vi "DefaultPersonality_5785_FPGA.vi"() -> ()   [LabVIEW 2018, in "GettingStarted_5785_FPGA.lvlib"]
uses:
  GettingStarted_5785_FPGA.lvlib
  <instrlib>/_niInstr/Streaming/v1/Common/Stream State.ctl
  <vilib>/Platform/TimedLoop/XDataNode/timing_clust.ctl
  <vilib>/Platform/TimedLoop/XDataNode/nitl_modes.ctl
  <vilib>/Platform/TimedLoop/XDataNode/wakeup.ctl
  <instrlib>/FlexRIO/DRAM FIFO/v2/FPGA/DRAM FIFO/FIFO Depth.ctl
  <instrlib>/FlexRIO/API/FPGA/v1/IO/NI5785/AO DSP Cfg.ctl
  Generation Engine Cfg.ctl
  DDC Cfg.ctl
  <vilib>/rvi/Emulation/niFpgaSctlEmulationGetInTimedLoop.vi
  <vilib>/rvi/Emulation/niFpgaEmulationReportErrorSimple.vi
  <vilib>/rvi/Emulation/niFpgaGetClockAttributes.vi
  <vilib>/rvi/Emulation/niFpgaCriticalErrorInLSC.vi
  <vilib>/rvi/eio/common/nirviEmuTemplateMethod_errors.vi
  <vilib>/rvi/DataTransferAndStorage/Container/Common/niFpgaContainerGetUniqueNameForEmu.vi
  <vilib>/rvi/DataTransferAndStorage/Container/Common/niFpgaContainerSetEmuInfo.vi
  <vilib>/rvi/eio/common/nirviEmuReportErrorAndStop.vi
  <vilib>/rvi/interface/RandomDataEmulation/nirviRandomDataMultiElementFPGAFIFO.vi
  <instcachedir>/0/nirviRandomDataMultiElementFPGAFIFO_6740B454F3C245F78F76ED91F73FD8DB.lvgen/nirviRandomDataMultiElementFPGAFIFO_6740B454F3C245F78F76ED91F73FD8DB_002.vi
  <vilib>/rvi/interface/RandomDataEmulation/niFpgaRandomDataHandleErrors.vi
  <vilib>/rvi/DataTransferAndStorage/Container/Common/niFpgaContainerExecOnDevCompGetState.vi
  <vilib>/rvi/Emulation/niFpgaEmulationIsFPGAContextNoSignature.vi
  <vilib>/rvi/errors/niFpgaSetErrorForExecOnDevCompSimple.vi
  <vilib>/rvi/FIFO/Fifo_Resource/nirvififoEmulationSetSize.vi
  <vilib>/rvi/FIFO/Fifo_Resource/nirviFifoEmulationQueueMgr.vi
  <instcachedir>/0/nirviFifoEmulationQueueMgr_E5CAEC123FF24DC58D834DCA3CDAA9B5.lvgen/nirviFifoEmulationQueueMgr_E5CAEC123FF24DC58D834DCA3CDAA9B5_015.vi
  <vilib>/rvi/FIFO/Fifo_Resource/nirvififoEmulationDetermineInputValidOut.vi
  <vilib>/rvi/FIFO/Fifo_Resource/nirvififoEmulationCreateLock.vi
  <vilib>/rvi/Emulation/niFpgaProcessEmulError.vi
  <vilib>/rvi/FIFO/Fifo_Resource/nirvififoEmulationObtainLock.vi
  <vilib>/rvi/FIFO/Fifo_Resource/nirvififoEmulationReleaseLock.vi
  <vilib>/rvi/occurrence/nirviWaitOnOccurrenceBase.vi
  <vilib>/rvi/errors/nirviReportUnexpectedCaseInternalError.vi
  <vilib>/rvi/errors/nirviReportUnexpectedCaseInternalError (U32).vi
  <vilib>/Utility/error.llb/Clear Errors.vi
  <instrlib>/FlexRIO/DRAM FIFO/v2/FPGA/DRAM FIFO/Private/DRAM FIFO U256x2/Create 256x2 DRAM FIFO.vi
  <instrlib>/_niInstr/Data Formatting/v1/FPGA/Private/Convert/Boolean Array to U16 Array.vi
  <vilib>/Platform/TimedLoop/XDataNode/XDataNode.xnode
  <vilib>/eio/EIONode/EIONode.xnode
  <vilib>/rvi/LocalResourceManager/LocalResourceManager.xnode
  <vilib>/rvi/DataTransferAndStorage/Container/XNode/niFpgaContainer.xnode
  <vilib>/rvi/interface/RandomDataEmulation/nirviRandomDataFpgaMultiElementTemplate.vi
  <vilib>/rvi/FIFO/Fifo_Resource/niFpgaFifoEmulationRefIn.vi
  <vilib>/rvi/DataTransferAndStorage/Handshake/Emulation/niFpgaHandshakeEmulationRefIn.vi
  <vilib>/Platform/TimedLoop/XDataNode/XDNodeRunTimeDep.lvlib
  <instrlib>/FlexRIO/API/FPGA/v1/FlexRIO API FPGA v1.lvlib
  <instrlib>/FlexRIO/DRAM FIFO/v2/FPGA/DRAM FIFO/DRAM FIFO v2 FPGA.lvclass
  <instrlib>/_niInstr/Data Formatting/v1/FPGA/niInstr Data Formatting v1 FPGA.lvlib
  <instrlib>/FlexRIO/API/FPGA/v1/IO/NI5785/FlexRIO 5785 FPGA v1.lvlib
  <instrlib>/_niInstr/Streaming/v1/Common/niInstr Streaming v1 Common.lvlib
  <instrlib>/FlexRIO/DRAM FIFO/v2/FPGA/DRAM FIFO/Private/DRAM FIFO U256x2/DRAM FIFO U256x2 v2 FPGA.lvclass
panel:
  in  "flexrio.dsp.reset 1":bool
  in  "flexrio.stream.channels enabled 1":u64
  out "flexrio.dsp.ready 1":bool
  in  "flexrio.stream.data.complex 1":bool
  in  "flexrio.dsp.duc.enable 1":bool
  in  "flexrio.dsp.duc.freq shift.mag 1.1":fxp<+/-,48,0>
  in  "flexrio.dsp.duc.freq shift.mag 1.0":fxp<+/-,48,0>
  in  "flexrio.dsp.ddc.enable 0":bool
  in  "flexrio.dsp.ddc.freq shift.mag 0.1":fxp<+/-,48,0>
  in  "flexrio.dsp.ddc.freq shift.mag 0.0":fxp<+/-,48,0>
  out "flexrio.dsp.ready 0":bool
  in  "flexrio.dsp.reset 0":bool
  in  "User-defined Start Trigger - AO":bool
  in  "flexrio.trigger.start.cfg 1":u16
  in  "flexrio.trigger.start.linked 1":bool
  out "flexrio.buffer.circular.written 1":u64
  out "flexrio.buffer.circular.size 1":u64
  in  "flexrio.io.interleaving factor 0":u16=1
  out "IO Socket\\AO Ready For Input":bool
  in  "stream.request state 1":T1
  in  "stream.num samples 1":u64
  out "stream.metadata 1":u64
  out "stream.samples transferred 1":u64
  out "stream.state 1":T1
  in  "flexrio.buffer.circular.reset 1":bool
  out "flexrio.module.dram ready 0":bool
  in  "flexrio.buffer.fifo.reset 0":bool
  out "flexrio.module.io ready 0":bool
  out "flexrio.module.io error 0":i32
  out "flexrio.module.data valid 0":bool
  in  "flexrio.stream.channels enabled 0":u64 caption="stream.num samples 0"
  in  "flexrio.buffer.delay.clocks 0":u16=1
  in  "flexrio.buffer.delay.reset 0":bool
  in  "flexrio.trigger.analog.edge.rising 0":bool=TRUE
  in  "flexrio.trigger.analog.edge.hysteresis 0":fxp<+/-,32,1>
  in  "flexrio.trigger.analog.edge.threshold 0":fxp<+/-,32,1>
  in  "User-defined Start Trigger - AI":bool
  in  "flexrio.trigger.start.cfg 0":u16
  in  "flexrio.trigger.analog.edge.channel 0":fxp<+,2,2> format="%#_4g"
  in  "stream.num samples 0":u64
  in  "stream.request state 0":T1
  out "stream.state 0":T1
  out "stream.samples transferred 0":u64
  out "stream.metadata 0":u64
  # "Data Path Configuration"
  # "AI Trigger Configuration"
  # "AI Stream Configuration"
  # "AO Stream Configuration"
  # "AI DSP Configuration"
  # "AO DSP Configuration"
  # "User-defined Controls"
  # "Module Status"
  # "AO Buffer Configuration"
  # "Device Utilization\n---------------------------\nTotal Slices: 86.1% (35694 out of 41460)\nSlice Registers: 31.8% (211112 out of 663360)\nSlice LUTs: 48.0% (159148 out of 331680)\nBlock RAMs: 40.5% (437 out of 1080)\nDSP48s: 32.1% (886 out of 2760)\n\nNote: Utilization numbers are for the KU060. Exact values will vary for other variants"
  # "AO Trigger Configuration"
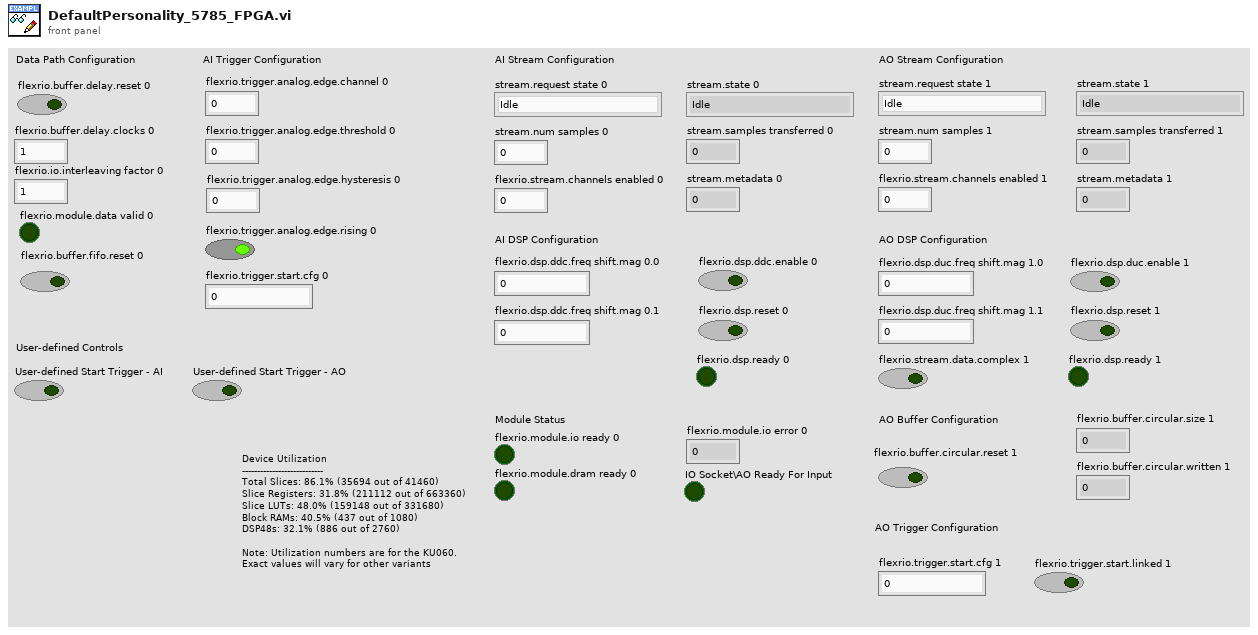
[diagram p1: front panel]
types:
  T1 = typedef "niInstr Streaming v1 Common.lvlib/Stream State.ctl" = enum8{"Idle", "Finite Transfer", "Continuous", "Done", "Error", "Not Ready", "Cancel"}
  T2 = typedef "XDNodeRunTimeDep.lvlib/timing_clust.ctl" = cluster{"Expected End [f-1]":u64, "Actual End [f-1]":u64, "Finished Late? [f-1]":bool, "Expected End [i-1]":u64, "Actual End [i-1]":u64, "Finished Late? [i-1]":bool, "Expected Start [i]":u64, "Actual Start [i]":u64, "Expected Start [f]":u64, "Actual Start [f]":u64, "Source Name":string, "Structure Name":string, "Period":i64, "Deadline":i64, "Offset":i64, "Start":i64, "Priority":i32, "Timeout":i32, "Mode":T3, "Wakeup Reason":T4, "Error":errorcluster, "Source Type":string, "Secondary Source Type":string, "Global End Time":u64, "Global Start Time":u64, "Frame Duration":u64, "Iteration Duration":u64, "Assigned CPU":i32, "I/O Scan Engine Mode":u32}
  T3 = typedef "XDNodeRunTimeDep.lvlib/nitl_modes.ctl" = enum32{"No Change", "Process missed periods, maintain original phase", "Discard missed periods, maintain original phase", "Process missed periods, ignore original phase", "Discard missed periods, ignore original phase"}
  T4 = typedef "XDNodeRunTimeDep.lvlib/wakeup.ctl" = enum32{"Normal", "Aborted", "Asynchronous wakeup", "Timing source error", "Timed loop error", "Timeout"}
  T5 = typedef "DRAM FIFO v2 FPGA.lvclass/FIFO Depth.ctl" = u8
  T6 = cluster{"flexrio.io.interleaving factor 0":u16, "flexrio.trigger.start.cfg 0":u16, "stream.num samples 0":u64, "stream.request state 0":T1, "flexrio.stream.channels enabled 0":u64, "flexrio.buffer.delay.clocks 0":u16, "flexrio.buffer.delay.reset 0":bool}
  T7 = typedef "GettingStarted_5785_FPGA.lvlib/DDC Cfg.ctl" = cluster{"flexrio.dsp.ddc.freq shift.mag 0.0":fxp<+/-,48,0>, "flexrio.dsp.ddc.freq shift.mag 0.1":fxp<+/-,48,0>, "flexrio.dsp.ddc.enable 0":bool, "flexrio.dsp.reset 0":bool}
  T8 = typedef "GettingStarted_5785_FPGA.lvlib/Generation Engine Cfg.ctl" = cluster{"flexrio.dsp.reset 1":bool, "flexrio.buffer.circular.reset 1":bool, "flexrio.stream.channels enabled 1":u64, "flexrio.trigger.start.linked 1":bool, "flexrio.trigger.start.cfg 1":u16, "stream.num samples 1":u64, "stream.request state 1":T1}
  T9 = cluster{"flexrio.trigger.analog.edge.channel 0":fxp<+,2,2>, "flexrio.trigger.analog.edge.threshold 0":fxp<+/-,32,1>, "flexrio.trigger.analog.edge.hysteresis 0":fxp<+/-,32,1>, "flexrio.trigger.analog.edge.rising 0":bool}
  T10 = typedef "FlexRIO 5785 FPGA v1.lvlib/AO DSP Cfg.ctl" = cluster{"flexrio.stream.data.complex 1":bool, "flexrio.dsp.duc.enable 1":bool, "flexrio.dsp.duc.freq shift.mag 1.0":fxp<+/-,48,0>, "flexrio.dsp.duc.freq shift.mag 1.1":fxp<+/-,48,0>}
  T11 = cluster{"stream.metadata 0":u64, "stream.samples transferred 0":u64, "stream.state 0":T1}
  T12 = cluster{"buffer size in elements":u64, "written elements":u64, "flexrio.dsp.ready 1":bool, "stream.metadata 1":u64, "stream.samples transferred 1":u64, "stream.state 1":T1}
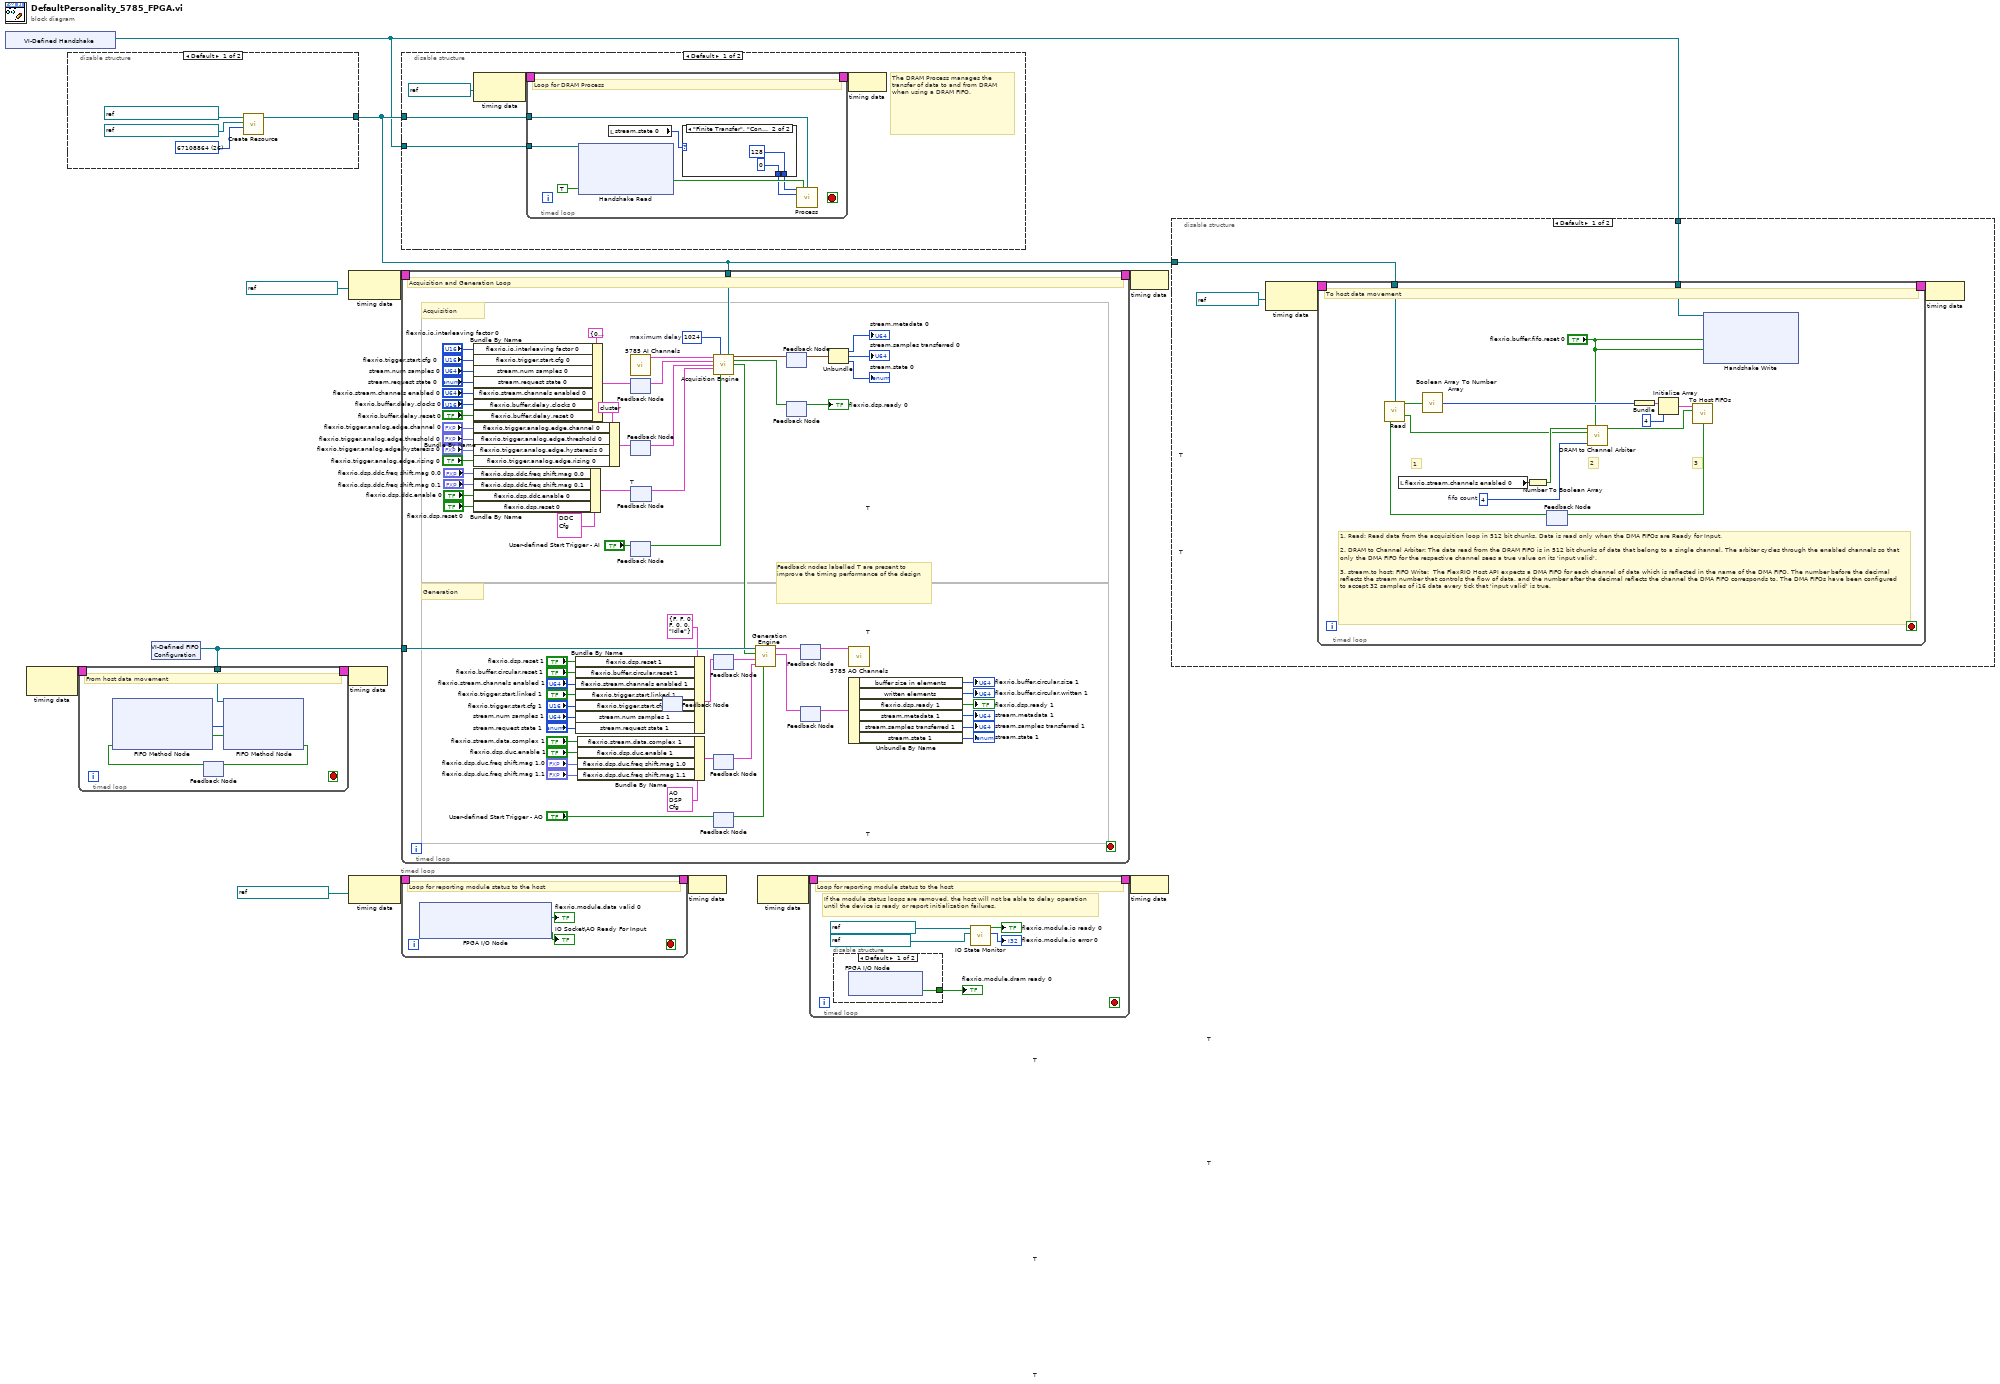
[diagram p0: block diagram]
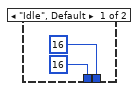
[diagram p3: hidden frame]
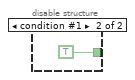
[diagram p6: hidden frame]
diagram:
  n1 = xnode "VI-Defined Handshake"() -> ("Handshake Out"=w7:refnum<k21>)
  n2 = node-c288() -> (w3:T2)  [unwired: 1 in]
  n3 = disable-structure shown="Default" {
    disable-tunnel: [w17 _] -> w8
    frame condition #0 (active) {
      w14 = T5 26 items=["4"=2, "8"=3, "16"=4, "32"=5, "64"=6, "128"=7, "256"=8, "512"=9, "1024"=10, "2048"=11, "4096"=12, "8192"=13, "16384"=14, "32768"=15, "65536"=16, "131072"=17, "262144"=18, "524288"=19, "1048576"=20, "2097152"=21, "4194304"=22, "8388608"=23, "16777216"=24, "33554432"=25, "67108864"=26, "134217728"=27, "268435456"=28, "536870912"=29, "1073741824"=30, "2147483648"=31, "4294967296"=32] ("actual # of DRAM elements")
      n4 = call-poly <instrlib>:"Create Resource.vi"("actual # of DRAM elements"=w14, "memory refnum 2"=refnum<k21> "DRAM FIFO Bank1 67108864" ("memory refnum"), "memory refnum"=refnum<k21> "DRAM FIFO Bank0 67108864") -> ("DRAM FIFO ref out"=w17:refnum<class "DRAM FIFO v2 FPGA.lvclass">)  [unwired: 8 in]
    }
    frame condition #1 {
    }
  }
  n5 = xnode "VI-Defined FIFO Configuration"() -> ("FIFO Out"=w1:refnum<k21>)
  n6 = timed-loop {
    timing: w3 -> [_]
    timing-out: [_] -> w2
    tunnel: w1 -> [w18]
    stop <- _ stop-if-true
    # "From host data movement"
    n7 = feedback #1() -> (w22:bool)  [unwired: 1 in]
    n8 = xnode ("FIFO Method Node")("Ready for Output"=w22) -> ("Element"=w19:i16[], "Output Valid"=w20:bool)  [unwired: 1 in, 1 out]
    n9 = xnode ("FIFO Method Node")("Element"=w19, "Input Valid"=w20, "FIFO In"=w18) -> ("Ready for Input"=w21:bool)  [unwired: 1 out]
    n10 = feedback-in #1(w21) -> ()
  }
  n11 = node-c288(refnum<k21> "IO Socket\\Data Clock" ("Source Name")) -> (w13:T2)
  n12 = node-c288(w2) -> ()
  n13 = node-c288(refnum<k21> "IO Socket\\Data Clock" ("Source Name")) -> (w6:T2)
  n14 = disable-structure shown="Default" {
    disable-tunnel: w8 -> [w26 _]
    disable-tunnel: w7 -> [w25 _]
    frame condition #0 (active) {
      # "The DRAM Process manages the transfer of data to and from DRAM when using a DRAM FIFO."
      n15 = node-c288(refnum<k21> "DRAM Clock" ("Source Name")) -> (w29:T2)
      n16 = timed-loop {
        timing: w29 -> [_]
        timing-out: [_] -> w28
        tunnel: w26 -> [w36]
        tunnel: w25 -> [w35]
        stop <- _ stop-if-true
        # "Loop for DRAM Process"
        n17 = xnode ("Handshake Read")("Ready for Output"=TRUE, "Handshake In"=w35) -> ("Output Valid"=w33:bool)  [unwired: 2 out]
        n18 = local read "stream.state 0"() -> (w32:T1)
        n19 = case shown="\"Finite Transfer\", \"Continuous\"" w32 {
          tunnel: [u16 16 ("write grant time (clock ticks)") u16 128 ("write grant time (clock ticks)")] -> w31
          tunnel: [u16 16 ("read grant time (clock ticks)") u16 0 ("read grant time (clock ticks)")] -> w30
          frame "Idle", Default {
          }
          frame "Finite Transfer", "Continuous" {
          }
        }
        n20 = call <instrlib>:"Process.vi"("write grant time (clock ticks)"=w31, "reset DRAM"=w33, "DRAM FIFO ref in"=w36, "read grant time (clock ticks)"=w30) -> ()  [unwired: 10 in, 2 out]
      }
      n21 = node-c288(w28) -> ()
    }
    frame condition #1 {
      # "The host can instruct the buffer to reset itself. To clear our all the data inside the FIFO the clear method is called. The clear method can only be accessed inside a while loop."
    }
  }
  n22 = timed-loop {
    timing: w13 -> [_]
    timing-out: [_] -> w12
    tunnel: w8 -> [w48]
    tunnel: w1 -> [w113]
    stop <- _ stop-if-true
    w47 = u16 1024  # maximum delay
    # "Feedback nodes labelled T are present to improve the timing performance of the design"
    # "Acquisition"
    # "Generation"
    # "Acquisition and Generation Loop"
    n23 = Bundle By Name(cluster=T6 {"flexrio.io.interleaving factor 0"=0, "flexrio.trigger.start.cfg 0"=0, "stream.num samples 0"=0, "stream.request state 0"=enum."Idle", "flexrio.stream.channels enabled 0"=0, "flexrio.buffer.delay.clocks 0"=0, "flexrio.buffer.delay.reset 0"=FALSE}, "flexrio.io.interleaving factor 0"="flexrio.io.interleaving factor 0", "flexrio.trigger.start.cfg 0"="flexrio.trigger.start.cfg 0", "stream.num samples 0"="stream.num samples 0", "stream.request state 0"="stream.request state 0", "flexrio.stream.channels enabled 0"="flexrio.stream.channels enabled 0", "flexrio.buffer.delay.clocks 0"="flexrio.buffer.delay.clocks 0", "flexrio.buffer.delay.reset 0"="flexrio.buffer.delay.reset 0") -> (w62:T6)
    n24 = Bundle By Name(cluster=T9 {"flexrio.trigger.analog.edge.channel 0"=0.0, "flexrio.trigger.analog.edge.threshold 0"=0.0, "flexrio.trigger.analog.edge.hysteresis 0"=0.0, "flexrio.trigger.analog.edge.rising 0"=FALSE}, "flexrio.trigger.analog.edge.channel 0"="flexrio.trigger.analog.edge.channel 0", "flexrio.trigger.analog.edge.threshold 0"="flexrio.trigger.analog.edge.threshold 0", "flexrio.trigger.analog.edge.hysteresis 0"="flexrio.trigger.analog.edge.hysteresis 0", "flexrio.trigger.analog.edge.rising 0"="flexrio.trigger.analog.edge.rising 0") -> (w55:T9)
    n25 = Bundle By Name(cluster=T7 {"flexrio.dsp.ddc.freq shift.mag 0.0"=0.0, "flexrio.dsp.ddc.freq shift.mag 0.1"=0.0, "flexrio.dsp.ddc.enable 0"=FALSE, "flexrio.dsp.reset 0"=FALSE}, "flexrio.dsp.ddc.freq shift.mag 0.0"="flexrio.dsp.ddc.freq shift.mag 0.0", "flexrio.dsp.ddc.freq shift.mag 0.1"="flexrio.dsp.ddc.freq shift.mag 0.1", "flexrio.dsp.ddc.enable 0"="flexrio.dsp.ddc.enable 0", "flexrio.dsp.reset 0"="flexrio.dsp.reset 0") -> (w105:T7)
    n26 = Bundle By Name(cluster=T8 {"flexrio.dsp.reset 1"=FALSE, "flexrio.buffer.circular.reset 1"=FALSE, "flexrio.stream.channels enabled 1"=0, "flexrio.trigger.start.linked 1"=FALSE, "flexrio.trigger.start.cfg 1"=0, "stream.num samples 1"=0, "stream.request state 1"=enum."Idle"} ("config in"), "flexrio.dsp.reset 1"="flexrio.dsp.reset 1", "flexrio.buffer.circular.reset 1"="flexrio.buffer.circular.reset 1", "flexrio.stream.channels enabled 1"="flexrio.stream.channels enabled 1", "flexrio.trigger.start.linked 1"="flexrio.trigger.start.linked 1", "flexrio.trigger.start.cfg 1"="flexrio.trigger.start.cfg 1", "stream.num samples 1"="stream.num samples 1", "stream.request state 1"="stream.request state 1") -> (w81:T8)
    n27 = Bundle By Name(cluster=T10 {"flexrio.stream.data.complex 1"=FALSE, "flexrio.dsp.duc.enable 1"=FALSE, "flexrio.dsp.duc.freq shift.mag 1.0"=0.0, "flexrio.dsp.duc.freq shift.mag 1.1"=0.0} ("dsp config"), "flexrio.stream.data.complex 1"="flexrio.stream.data.complex 1", "flexrio.dsp.duc.enable 1"="flexrio.dsp.duc.enable 1", "flexrio.dsp.duc.freq shift.mag 1.0"="flexrio.dsp.duc.freq shift.mag 1.0", "flexrio.dsp.duc.freq shift.mag 1.1"="flexrio.dsp.duc.freq shift.mag 1.1") -> (w70:T10)
    n28 = call <instrlib>:"5785 AI Channels.vi"() -> ("all channels"=w57:cluster{fxp<+/-,12,1>[]}[])  [unwired: 15 in]
    n29 = feedback-in #2(w62) -> ()
    n30 = feedback #2 "T"() -> (w56:T6)  [unwired: 1 in]
    n31 = feedback-in #3(w55) -> ()
    n32 = feedback #3 "T"() -> (w54:T9)  [unwired: 1 in]
    n33 = feedback-in #4("User-defined Start Trigger - AI") -> ()
    n34 = feedback #4 "T"() -> (w49:bool)  [unwired: 1 in]
    n35 = feedback #5 "T"() -> (w53:T7)  [unwired: 1 in]
    n36 = feedback-in #5(w105) -> ()
    n37 = feedback-in #6(w81) -> ()
    n38 = feedback #6() -> (w71:T8)  [unwired: 1 in]
    n39 = call "Acquisition Engine.vi"("all channels"=w57, "delay buffer size"=w47, "DRAM FIFO v2 FPGA in"=w48, "streaming control"=w56, "analog trigger"=w54, "ddc dsp"=w53, "User-defined Start Trigger - AI"=w49) -> ("streaming indicators"=w111:T11, "flexrio.dsp.ready 0"=w112:bool, "start trigger to AO"=w67:bool)  [unwired: 6 in]
    n40 = feedback-in #7(w71) -> ()
    n41 = feedback #7 "T"() -> (w69:T8)  [unwired: 1 in]
    n42 = feedback-in #8(w70) -> ()
    n43 = feedback #8 "T"() -> (w68:T10)  [unwired: 1 in]
    n44 = feedback-in #9("User-defined Start Trigger - AO") -> ()
    n45 = feedback #9 "T"() -> (w80:bool)  [unwired: 1 in]
    n46 = call "Generation Engine.vi"("User-defined Start Trigger - AO"=w80, "dsp config"=w68, "config in"=w69, "linked start trigger from ai"=w67, "fifo from host"=w113) -> ("state out"=w83:T12, "data to IO node"=w99:cluster{"ao1":fxp<+/-,12,1>[]}[])  [unwired: 5 in]
    n47 = feedback #10 "T"() -> (w110:T11)  [unwired: 1 in]
    n48 = feedback-in #10(w111) -> ()
    n49 = feedback-in #11(w112) -> ()
    n50 = feedback #11 "T"() -> (→"flexrio.dsp.ready 0":bool)  [unwired: 1 in]
    n51 = feedback #12 "T"() -> (w98:cluster{"ao1":fxp<+/-,12,1>[]}[])  [unwired: 1 in]
    n52 = feedback-in #12(w99) -> ()
    n53 = feedback-in #13(w83) -> ()
    n54 = feedback #13 "T"() -> (w79:T12)  [unwired: 1 in]
    n55 = Unbundle(w110) -> ("stream.metadata 0"=→"stream.metadata 0":u64, "stream.samples transferred 0"=→"stream.samples transferred 0":u64, "stream.state 0"=→"stream.state 0":T1)
    n56 = call <instrlib>:"5785 AO Channels.vi"("all channels"=w98) -> ()  [unwired: 15 in]
    n57 = Unbundle By Name(w79) -> ("buffer size in elements"=→"flexrio.buffer.circular.size 1":u64, "written elements"=→"flexrio.buffer.circular.written 1":u64, "flexrio.dsp.ready 1"=→"flexrio.dsp.ready 1":bool, "stream.metadata 1"=→"stream.metadata 1":u64, "stream.samples transferred 1"=→"stream.samples transferred 1":u64, "stream.state 1"=→"stream.state 1":T1)
  }
  n58 = timed-loop {
    timing: w6 -> [_]
    timing-out: [_] -> w5
    stop <- _ stop-if-true
    # "Loop for reporting module status to the host"
    n59 = xnode "FPGA I/O Node"() -> ("IO Socket\\AI Data Valid"=→"flexrio.module.data valid 0":bool, "IO Socket\\AO Ready For Input"=→"IO Socket\\AO Ready For Input":bool)  [unwired: 2 in, 2 out]
  }
  n60 = node-c288(w5) -> ()
  n61 = node-c288() -> (w10:T2)  [unwired: 1 in]
  n62 = timed-loop {
    timing: w10 -> [_]
    timing-out: [_] -> w9
    stop <- _ stop-if-true
    # "If the module status loops are removed, the host will not be able to delay operation until the device is ready or report initialization failures."
    # "Loop for reporting module status to the host"
    n63 = disable-structure shown="Default" {
      disable-tunnel: [w126 TRUE ("flexrio.module.dram ready 0")] -> w123
      frame condition #0 (active) {
        n64 = xnode "FPGA I/O Node"() -> ("DRAM Ready"=w126:bool)  [unwired: 1 in, 1 out]
      }
      frame condition #1 {
      }
    }
    "flexrio.module.dram ready 0" <- w123
    n65 = call <instrlib>:"IO State Monitor.vi"("io error resource"=refnum<k21> "IO Socket\\IO Error" ("FPGA I/O In"), "io ready resource"=refnum<k21> "IO Socket\\IO Ready" ("FPGA I/O In")) -> ("flexrio.module.io error 0"=→"flexrio.module.io error 0":i32, "flexrio.module.io ready 0"=→"flexrio.module.io ready 0":bool)  [unwired: 8 in]
  }
  n66 = node-c288(w12) -> ()
  n67 = node-c288(w9) -> ()
  n68 = disable-structure shown="Default" {
    disable-tunnel: w8 -> [w131 _]
    disable-tunnel: w7 -> [w130 _]
    frame condition #0 (active) {
      n69 = node-c288(refnum<k21> "PXIe_CLK200" ("Source Name")) -> (w134:T2)
      n70 = timed-loop {
        timing: w134 -> [_]
        timing-out: [_] -> w133
        tunnel: w131 -> [w148]
        tunnel: w130 -> [w146]
        stop <- _ stop-if-true
        w143 = 4  # fifo count
        # "3"
        # "2"
        # "1. Read: Read data from the acquisition loop in 512 bit chunks. Data is read only when the DMA FIFOs are Ready for Input.\n\n2. DRAM to Channel Arbiter: The data read from the DRAM FIFO is in 512 bit chunks of data that belong to a single channel. The arbiter cycles through the enabled channels so that only the DMA FIFO for the respective channel sees a true value on its 'input valid'. \n\n3. stream.to host: FIFO Write:  The FlexRIO Host API expects a DMA FIFO for each channel of data which is reflected in the name of the DMA FIFO. The number before the decimal reflects the stream number that controls the flow of data, and the number after the decimal reflects the channel the DMA FIFO corresponds to. The DMA FIFOs have been configured to accept 32 samples of i16 data every tick that 'input valid' is true."
        # "1"
        # "To host data movement"
        n71 = local read "flexrio.stream.channels enabled 0"() -> (w149:u64)
        n72 = Number To Boolean Array(number=w149) -> (Boolean array=w145:bool[])
        n73 = feedback #14() -> (w136:bool)  [unwired: 1 in]
        n74 = call <instrlib>:"Read.vi"("DRAM FIFO ref in"=w148, "ready for output"=w136) -> ("element"=w135:bool[], "output valid"=w144:bool)  [unwired: 12 in]
        n75 = call-poly <instrlib>:"Boolean Array To Number Array.vi"("data in"=w135) -> ("data out"=w147:u16[])  [unwired: 14 in]
        n76 = call <instrlib>:"DRAM to Channel Arbiter.vi"("reset"="flexrio.buffer.fifo.reset 0", "channel count"=w143, "input valid"=w144, "channels enabled"=w145) -> ("valid channel"=w138:bool[])  [unwired: 6 in, 1 out]
        n77 = Bundle("data out"=w147) -> (w141:cluster{"data out":u16[]})  [unwired: 1 in]
        n78 = Initialize Array(w141, 4 ("dimension size")) -> (w139:cluster{"data out":u16[]}[])
        n79 = call "To Host FIFOs.vi"("data"=w139, "data valid"=w138) -> ("all ready for input"=w137:bool)  [unwired: 12 in, 1 out]
        n80 = feedback-in #14(w137) -> ()
        n81 = xnode ("Handshake Write")("Data"="flexrio.buffer.fifo.reset 0", "Input Valid"="flexrio.buffer.fifo.reset 0", "Handshake In"=w146) -> ()  [unwired: 2 out]
      }
      n82 = node-c288(w133) -> ()
    }
    frame condition #1 {
    }
  }
